vi "Get name from label (Sub-diagnostics).vi"(7 "SMEnqueuer":refnum<class "Message Enqueuer.lvclass">, 8 "error in":errorcluster, 9 "Current diagnostics":string, 10 "Selected label":string, 11 "UI JSON read cluster":T1={"UIParameters"={"SpecificationVersion"="", "Title"="", "NumberOfImagesToBeDisplayed"=1.0, "ImageCountWindow"=1.0, "FontName"="", "FontSize"=2.0, "CustomerLogoFilePath"="", "ZentronLogoFilePath"="", "CompatibleSoftwareVersions"=[], "CameraLabelMapping"=[], "ImageIndicatorLayouts"=[], "SoftwareButtonLabels"={"SelectLabel"="", "RunLabel"="", "PauseLabel"="", "StopLabel"=""}, "DiagnosticsParameters"={"CameraOpticsDiagnostics"={"Label"="", "CameraLabelsList"=[]}, "ArduinoDiagnostics"={"Label"=""}, "MotorDiagnostics"={"Label"=""}, "ReelerMotor"={"Label"=""}, "TowerLampDiagnostics"={"Label"=""}, "TriggerSensor"={"Label"="", "SensorsList"=[]}, "HardwareButtonDiagnostics"={"Label"=""}, "MasterSampleDiagnostics"={"Label"=""}}, "DieIdParameters"={"DefaultDieId"="", "DieIdsList"=[]}, "EventReasonsList"={"Pause"=[], "Stop"=[], "FailPause"=[], "Ignored"=[], "DefaultEventReason"=""}, "StampingMachineIds"=[], "ErrorPopupStrings"=[]}}) -> (0 "error out":errorcluster, 3 "Diagnostics name":string)   [LabVIEW 2019, in "ZenGage v3.0 UI.lvclass"]
uses:
  ZenGage v3.0 UI.lvclass
  <vilib>/ActorFramework/Message Enqueuer/Message Enqueuer.lvclass
  Common/Controls/Acknowledgement.ctl
  Type Definitions/General/OutputDetails.ctl
  Type Definitions/General/Output choice.ctl
  Type Definitions/JSON Read/UI JSON read cluster.ctl
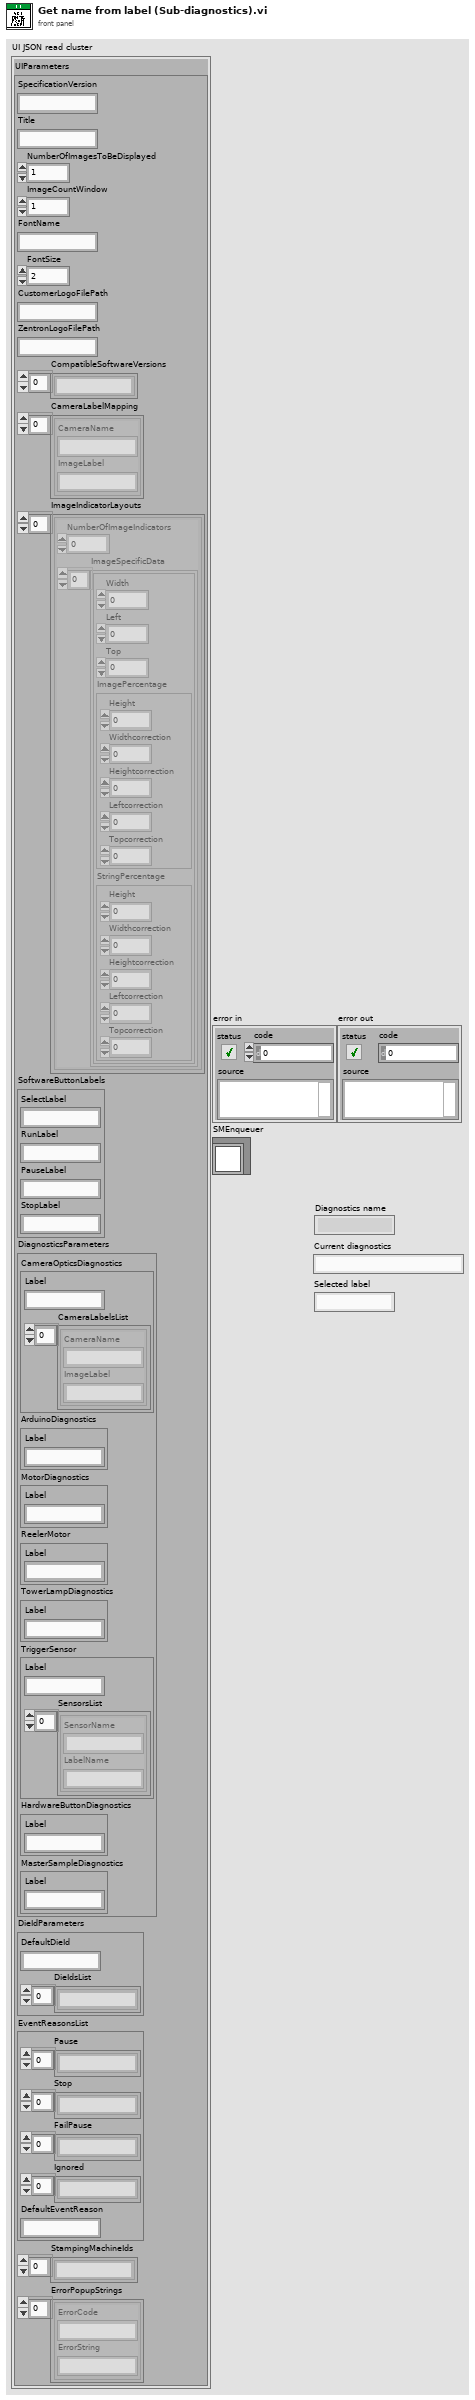
[diagram p1: front panel]
types:
  T1 = typedef "ZenGage v3.0 UI.lvclass/UI JSON read cluster.ctl" = cluster{"UIParameters":cluster{"SpecificationVersion":string, "Title":string, "NumberOfImagesToBeDisplayed":dbl, "ImageCountWindow":dbl, "FontName":string, "FontSize":dbl, "CustomerLogoFilePath":string, "ZentronLogoFilePath":string, "CompatibleSoftwareVersions":string[], "CameraLabelMapping":cluster{"CameraName":string, "ImageLabel":string}[], "ImageIndicatorLayouts":cluster{"NumberOfImageIndicators":dbl, "ImageSpecificData":cluster{"Width":dbl, "Left":dbl, "Top":dbl, "ImagePercentage":cluster{"Height":dbl, "Widthcorrection":i64, "Heightcorrection":i64, "Leftcorrection":dbl, "Topcorrection":dbl}, "StringPercentage":cluster{"Height":dbl, "Widthcorrection":i64, "Heightcorrection":dbl, "Leftcorrection":dbl, "Topcorrection":dbl}}[]}[], "SoftwareButtonLabels":cluster{"SelectLabel":string, "RunLabel":string, "PauseLabel":string, "StopLabel":string}, "DiagnosticsParameters":cluster{"CameraOpticsDiagnostics":cluster{"Label":string, "CameraLabelsList":cluster{"CameraName":string, "ImageLabel":string}[]}, "ArduinoDiagnostics":cluster{"Label":string}, "MotorDiagnostics":cluster{"Label":string}, "ReelerMotor":cluster{"Label":string}, "TowerLampDiagnostics":cluster{"Label":string}, "TriggerSensor":cluster{"Label":string, "SensorsList":cluster{"SensorName":string, "LabelName":string}[]}, "HardwareButtonDiagnostics":cluster{"Label":string}, "MasterSampleDiagnostics":cluster{"Label":string}}, "DieIdParameters":cluster{"DefaultDieId":string, "DieIdsList":string[]}, "EventReasonsList":cluster{"Pause":string[], "Stop":string[], "FailPause":string[], "Ignored":string[], "DefaultEventReason":string}, "StampingMachineIds":string[], "ErrorPopupStrings":cluster{"ErrorCode":string, "ErrorString":string}[]}}
  T2 = cluster{"CameraOpticsDiagnostics":cluster{"Label":string, "CameraLabelsList":cluster{"CameraName":string, "ImageLabel":string}[]}, "ArduinoDiagnostics":cluster{"Label":string}, "MotorDiagnostics":cluster{"Label":string}, "ReelerMotor":cluster{"Label":string}, "TowerLampDiagnostics":cluster{"Label":string}, "TriggerSensor":cluster{"Label":string, "SensorsList":cluster{"SensorName":string, "LabelName":string}[]}, "HardwareButtonDiagnostics":cluster{"Label":string}, "MasterSampleDiagnostics":cluster{"Label":string}}
  T3 = typedef "ZenGage v3.0 UI.lvclass/Output choice.ctl" = enum16{"SendIgnoredFailCount", "SendPartDetails", "ButtonPress", "SendAcknowledgement", "InitiateCameraDiagnostics", "InitiateSensorDiagnostics", "SendPopupResponse", "SendEventReasonResponse", "SendErrorDetails"}
  T4 = typedef "ZenGage v3.0 UI.lvclass/OutputDetails.ctl" = cluster{"Acknowledgement_SM":T5, "Button name":string, "PartDetails":cluster{"PartName":string, "ConnectorsInReel":u64, "TotalCounts":u64, "OperatorName":string, "StampingMachineID":u32}, "SensorName":string, "CameraName":string, "PopupFeedbackDetails":cluster{"Pop-up Type":enum16{"Open Logo Display", "Close Logo Display", "Open Loading Bar", "Close Loading Bar", "Open Alert Display", "Close Alert Display", "One button dialog box", "Two button dialog box", "User Authentication"}, "Message":string, "Pressed Button":string}, "EventResponse":string, "ErrorMessage":string, "FailCountIgnore":cluster{"ReelIgnoreCount":u64, "ProductionIgnoreCount":u64}}
  T5 = typedef "Acknowledgement.ctl" = cluster{"Enqueuer":refnum<class "Message Enqueuer.lvclass">, "VIReference":refnum<vi>, "VIName":string}
  T6 = cluster{"SensorName":string, "LabelName":string}[]
  T7 = cluster{"CameraName":string, "ImageLabel":string}[]
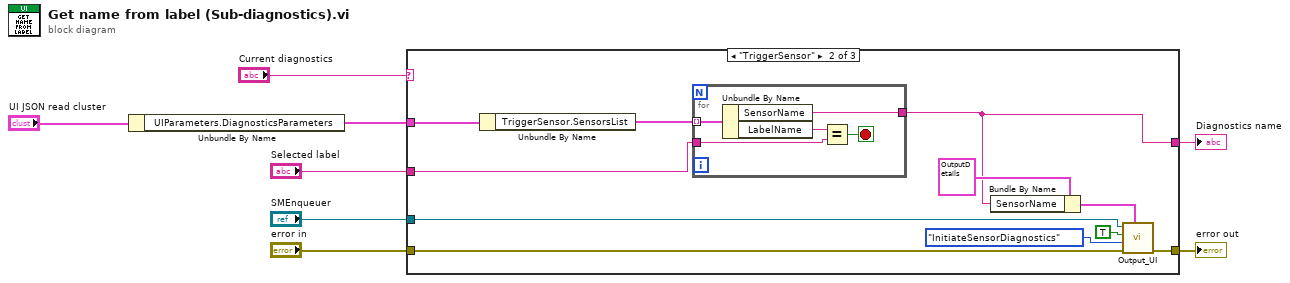
[diagram p0: block diagram]
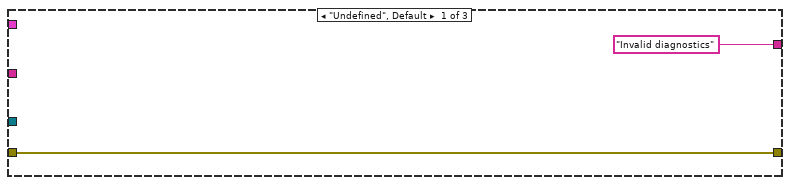
[diagram p2: hidden frame]
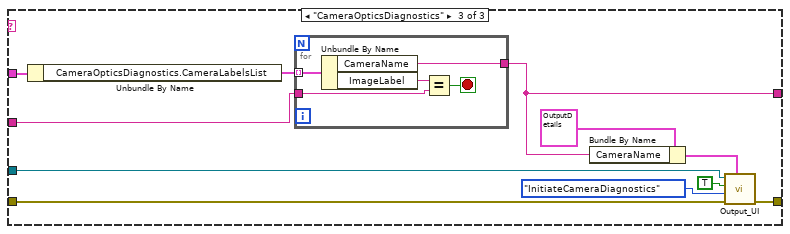
[diagram p3: hidden frame]
diagram:
  n1 = Unbundle By Name("UI JSON read cluster") -> ("UIParameters.DiagnosticsParameters"=w6:T2)
  n2 = case shown="\"TriggerSensor\"" "Current diagnostics" {
    tunnel: w6 -> [_ w21 w37]
    tunnel: "Selected label" -> [_ w19 w35]
    tunnel: ["Invalid diagnostics" ("SensorName") w13 w29] -> w4
    tunnel: "error in" -> [w9 w14 w31]
    tunnel: [w9 w15 w30] -> w2
    tunnel: "SMEnqueuer" -> [_ w12 w28]
    frame "Undefined", Default {
    }
    frame "TriggerSensor" {
      n3 = Unbundle By Name(w21) -> ("TriggerSensor.SensorsList"=w20:T6)
      n4 = for {
        tunnel: w20 -> [w26] mode=indexing
        tunnel: w19 -> [w24]
        tunnel: [w22] -> w13
        stop <- w23 stop-if-true
        n5 = Unbundle By Name(w26) -> ("SensorName"=w22:string, "LabelName"=w25:string)
        n6 = Equal?(x=w25, y=w24) -> (x = y?=w23:bool)
      }
      n7 = Bundle By Name(cluster=T4 {"Acknowledgement_SM"={"Enqueuer"=refnum, "VIReference"=refnum, "VIName"=""}, "Button name"="", "PartDetails"={"PartName"="", "ConnectorsInReel"=0, "TotalCounts"=0, "OperatorName"="", "StampingMachineID"=0}, "SensorName"="", "CameraName"="", "PopupFeedbackDetails"={"Pop-up Type"=enum."Open Logo Display", "Message"="", "Pressed Button"=""}, "EventResponse"="", "ErrorMessage"="", "FailCountIgnore"={"ReelIgnoreCount"=0, "ProductionIgnoreCount"=0}} ("OutputDetails"), "SensorName"=w13) -> (w16:T4)
      n8 = call "Output_UI.vi"("OutputDetails"=w16, "error in"=w14, "Functionality"=Output_choice."InitiateSensorDiagnostics", "Testbench"=TRUE, "SMEnqueuer"=w12) -> ("error out"=w15:errorcluster)  [unwired: 6 in]
    }
    frame "CameraOpticsDiagnostics" {
      n9 = Unbundle By Name(w37) -> ("CameraOpticsDiagnostics.CameraLabelsList"=w36:T7)
      n10 = for {
        tunnel: w36 -> [w42] mode=indexing
        tunnel: w35 -> [w40]
        tunnel: [w38] -> w29
        stop <- w39 stop-if-true
        n11 = Unbundle By Name(w42) -> ("CameraName"=w38:string, "ImageLabel"=w41:string)
        n12 = Equal?(x=w41, y=w40) -> (x = y?=w39:bool)
      }
      n13 = Bundle By Name(cluster=T4 {"Acknowledgement_SM"={"Enqueuer"=refnum, "VIReference"=refnum, "VIName"=""}, "Button name"="", "PartDetails"={"PartName"="", "ConnectorsInReel"=0, "TotalCounts"=0, "OperatorName"="", "StampingMachineID"=0}, "SensorName"="", "CameraName"="", "PopupFeedbackDetails"={"Pop-up Type"=enum."Open Logo Display", "Message"="", "Pressed Button"=""}, "EventResponse"="", "ErrorMessage"="", "FailCountIgnore"={"ReelIgnoreCount"=0, "ProductionIgnoreCount"=0}} ("OutputDetails"), "CameraName"=w29) -> (w32:T4)
      n14 = call "Output_UI.vi"("OutputDetails"=w32, "error in"=w31, "Functionality"=Output_choice."InitiateCameraDiagnostics", "Testbench"=TRUE, "SMEnqueuer"=w28) -> ("error out"=w30:errorcluster)  [unwired: 6 in]
    }
  }
  "Diagnostics name" <- w4
  "error out" <- w2
